vi "VISA write.vi"(8 "error in (no error)":errorcluster, 11 "Cobolt in":refnum<class "Cobolt.lvclass">) -> (0 "error out":errorcluster, 3 "Cobolt out":refnum<class "Cobolt.lvclass">)   [LabVIEW 2012, in "Cobolt.lvclass"]
uses:
  Cobolt.lvclass
panel:
  out "concatenated string":string
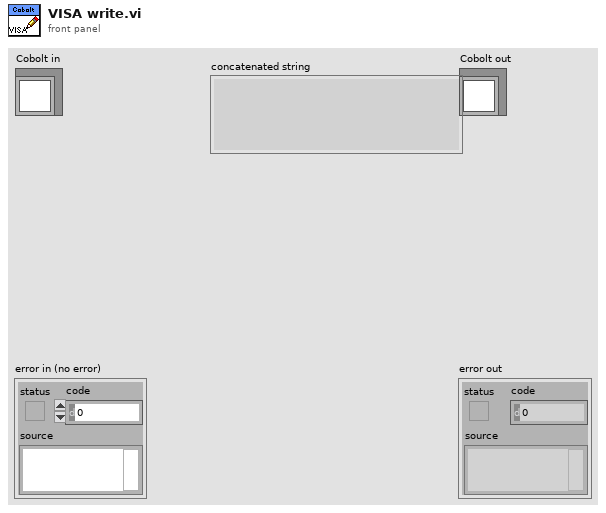
[diagram p1: front panel]
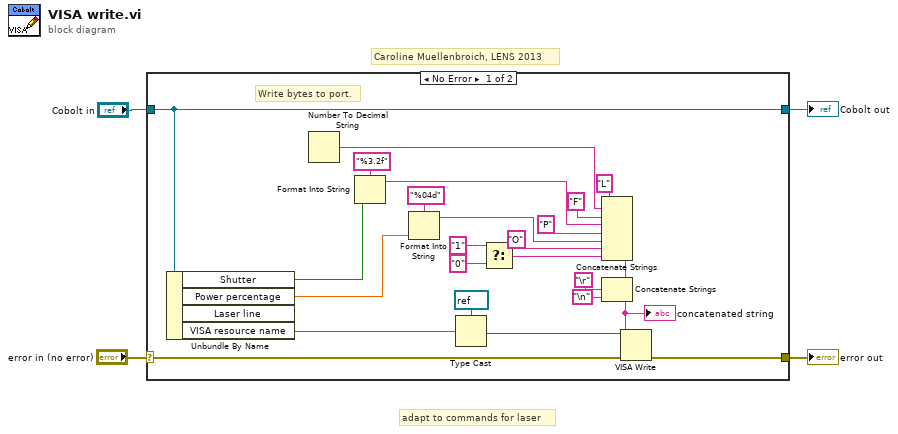
[diagram p0: block diagram]
diagram:
  # "adapt to commands for laser"
  # "Caroline Muellenbroich, LENS 2013"
  n1 = case shown="No Error" "error in (no error)" {
    selector: "error in (no error)" -> [w6 w30]
    tunnel: [w5 w30] -> w3
    tunnel: [w7 w29] -> w1
    tunnel: "Cobolt in" -> [w7 w29]
    frame No Error {
      # "Write bytes to port."
      n2 = Unbundle By Name(w7) -> ("Shutter"=w20:bool, "Power percentage"=w23:dbl, "VISA resource name"=w16:string)  [unwired: 1 out]
      n3 = Number To Decimal String() -> (decimal integer string=w18:string)  [unwired: 2 in]
      n4 = Format Into String(format string="%3.2f", w20) -> (resulting string=w22:string)  [unwired: 2 in, 1 out]
      n5 = Format Into String(format string="%04d", w23) -> (resulting string=w24:string)  [unwired: 2 in, 1 out]
      n6 = Type Cast(type=refnum<visa-resource-name> refnum ("VISA resource name"), x=w16) -> (*(type *) &x=w19:refnum<visa-resource-name>)
      n7 = Select(t="1" ("string"), f="0" ("string")) -> (s? t:f=w26:string)  [unwired: 1 in]
      n8 = Concatenate Strings("L", w18, "F" ("string"), w22, "P" ("string"), w24, "O" ("string"), w26) -> (w8:string)
      n9 = Concatenate Strings(w8, "\r", "\n") -> (w14:string)
      "concatenated string" <- w14
      n10 = VISA Write(VISA resource name=w19, write buffer=w14, error in (no error)=w6) -> (error out=w5:errorcluster)  [unwired: 2 out]
    }
    frame Error {
    }
  }
  "error out" <- w3
  "Cobolt out" <- w1
